vi "Create Payload (Constant).vi"(7 "Bit Length":u16(ring) items=["Byte (8 bits)", "Word (16 bits)", "Long (32 bits)", "Quad (64 bits)"], 10 "Value":u64 format="%.0x", 11 "Length":i32) -> (2 "Value not in range?":bool, 3 "Payload (U8)":u8[](array[numeric]) format="%.0x")   [LabVIEW 2020, in "EthFrameManagement.lvlib"]
uses:
  EthFrameManagement.lvlib
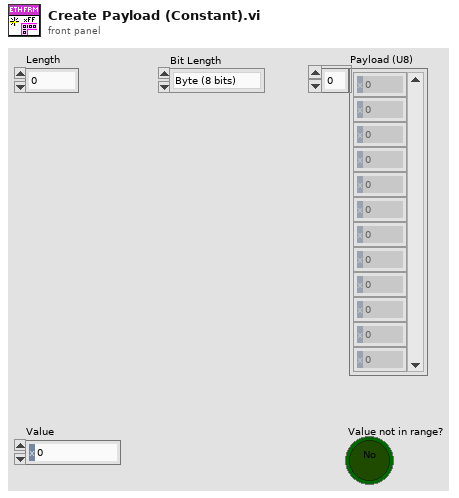
[diagram p1: front panel]
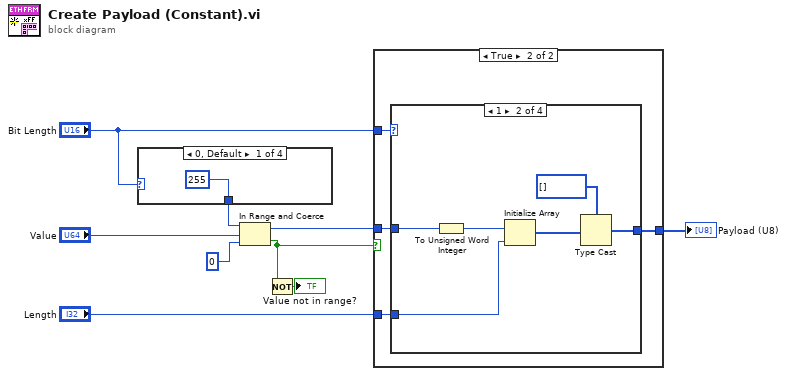
[diagram p0: block diagram]
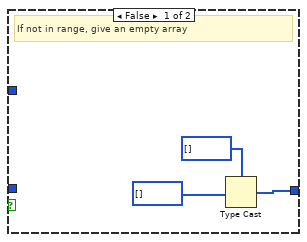
[diagram p2: hidden frame]
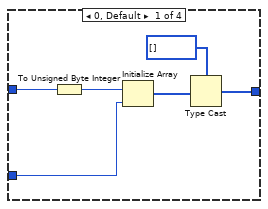
[diagram p3: hidden frame]
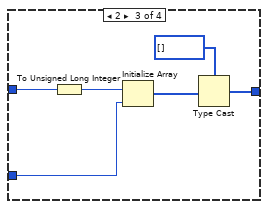
[diagram p4: hidden frame]
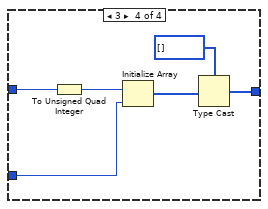
[diagram p5: hidden frame]
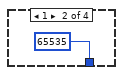
[diagram p6: hidden frame]
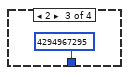
[diagram p7: hidden frame]
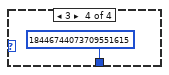
[diagram p8: hidden frame]
diagram:
  n1 = case shown="0, Default" "Bit Length" {
    tunnel: [u64 255 ("upper limit") u64 65535 ("upper limit") u64 4294967295 ("upper limit") u64 18446744073709551615 ("upper limit")] -> w7
    frame 0, Default {
    }
    frame 1 {
    }
    frame 2 {
    }
    frame 3 {
    }
  }
  n2 = In Range and Coerce(upper limit=w7, x="Value", lower limit=u64 0) -> (coerced(x)=w5:u64, In Range?=w3:bool)
  n3 = Not(x=w3) -> (.not. x?=→"Value not in range?":bool)
  n4 = case shown="True" w3 {
    tunnel: "Bit Length" -> [_ w20]
    tunnel: w5 -> [_ w19]
    tunnel: "Length" -> [_ w18]
    tunnel: [w15 w17] -> w2
    frame False {
      # "If not in range, give an empty array"
      n5 = Type Cast(type=u8[] [] ("Array"), x=u8[] [] ("Array")) -> (*(type *) &x=w15:u8[])
    }
    frame True {
      n6 = case shown="1" w20 {
        tunnel: w19 -> [w25 w31 w37 w43]
        tunnel: w18 -> [w26 w32 w38 w44]
        tunnel: [w21 w27 w33 w39] -> w17
        frame 0, Default {
          n7 = To Unsigned Byte Integer(number=w25) -> (unsigned 8bit integer=w24:u8)
          n8 = Initialize Array(w24, w26) -> (w22:u8[])
          n9 = Type Cast(type=u8[] [] ("Array"), x=w22) -> (*(type *) &x=w21:u8[])
        }
        frame 1 {
          n10 = To Unsigned Word Integer(number=w31) -> (unsigned 16bit integer=w30:u16)
          n11 = Initialize Array(w30, w32) -> (w28:u16[])
          n12 = Type Cast(type=u8[] [] ("Array"), x=w28) -> (*(type *) &x=w27:u8[])
        }
        frame 2 {
          n13 = To Unsigned Long Integer(number=w37) -> (unsigned 32bit integer=w36:u32)
          n14 = Initialize Array(w36, w38) -> (w34:u32[])
          n15 = Type Cast(type=u8[] [] ("Array"), x=w34) -> (*(type *) &x=w33:u8[])
        }
        frame 3 {
          n16 = To Unsigned Quad Integer(1:w43) -> (0:w42:u64)
          n17 = Initialize Array(w42, w44) -> (w40:u64[])
          n18 = Type Cast(type=u8[] [] ("Array"), x=w40) -> (*(type *) &x=w39:u8[])
        }
      }
    }
  }
  "Payload (U8)" <- w2
